vi "ADAM 5000 Get Voltages Manny.vi"(8 "error in (no error)":errorcluster, 10 "AI Sensor Data":T1={"Sensor Array"=[{"Description"="PT LOX Tank", "Last Reading"="1.37", "Coefs"=[0.0, 0.0], "Eng Units"="Psig"}, {"Description"="P3 - Fuel Tank Pressure", "Last Reading"="0.24", "Coefs"=[0.0, 5000.0], "Eng Units"="psig"}, {"Description"="P1 - Chamber Pressure", "Last Reading"="68.57", "Coefs"=[0.0, 5000.0], "Eng Units"="psig"}, {"Description"="Not Used", "Last Reading"="88.17", "Coefs"=[0.0, 0.0], "Eng Units"="psig"}, {"Description"="P5- DOME Reg.", "Last Reading"="1995.18", "Coefs"=[0.0, 5000.0], "Eng Units"="psig"}, {"Description"="Not Use", "Last Reading"="30.30", "Coefs"=[0.0, 0.0], "Eng Units"="psig"}, {"Description"="P4- High Pressure Tank", "Last Reading"="45.96", "Coefs"=[0.0, 10000.0], "Eng Units"="psig"}, {"Description"="P7 - Gnd High Pressure", "Last Reading"="1989.04", "Coefs"=[0.0, 10000.0], "Eng Units"="psig"}, {"Description"="P6 - GHE Fill Pressure", "Last Reading"="9918.82", "Coefs"=[0.0, 5000.0], "Eng Units"="psig"}, {"Description"="P8 - Pneumatics Pressure", "Last Reading"="9988.56", "Coefs"=[0.0, 5000.0], "Eng Units"="psig"}, {"Description"="Not Used", "Last Reading"="9997.25", "Coefs"=[0.0, 0.0], "Eng Units"=""}, {"Description"="Not Used", "Last Reading"="9988.56", "Coefs"=[0.0, 0.0], "Eng Units"=""}, {"Description"="Not Used", "Last Reading"="9948.58", "Coefs"=[0.0, 0.0], "Eng Units"=""}, {"Description"="Not Used", "Last Reading"="9973.45", "Coefs"=[0.0, 0.0], "Eng Units"=""}, {"Description"="Not Used", "Last Reading"="9964.45", "Coefs"=[0.0, 0.0], "Eng Units"=""}, {"Description"="PT High Press", "Last Reading"="9.16", "Coefs"=[0.0, 0.0], "Eng Units"="Psig"}, {"Description"="QD Sep Indication", "Last Reading"="2374.97", "Coefs"=[0.0, 1.0], "Eng Units"="On/Off"}, {"Description"="Lift Off Indicator", "Last Reading"="2375.24", "Coefs"=[0.0, 1.0], "Eng Units"="On/Off"}, {"Description"="Main Valve Open Indicator", "Last Reading"="2376.46", "Coefs"=[0.0, 1.0], "Eng Units"="On/Off"}, {"Description"="Main Valve Closed Indicator", "Last Reading"="2376.23", "Coefs"=[0.0, 1.0], "Eng Units"="On/Off"}, {"Description"="Load Cell 1 - Veh Gross Weight", "Last Reading"="2374.97", "Coefs"=[-122.0, 8333.3], "Eng Units"="lbf"}, {"Description"="Load Cell 2 - - Veh Gross Weight", "Last Reading"="2374.97", "Coefs"=[0.0, 8333.33], "Eng Units"="lbf"}, {"Description"="Not Used", "Last Reading"="2374.97", "Coefs"=[0.0, 0.0], "Eng Units"=""}, {"Description"="Not Used", "Last Reading"="2374.97", "Coefs"=[0.0, 0.0], "Eng Units"=""}, {"Description"="PT Fuel Tank", "Last Reading"="10.72", "Coefs"=[], "Eng Units"="Psig"}, {"Description"="", "Last Reading"="2401.98", "Coefs"=[], "Eng Units"=""}, {"Description"="PT Dome Set", "Last Reading"="0", "Coefs"=[], "Eng Units"="Psig"}, {"Description"="", "Last Reading"="2402.71", "Coefs"=[], "Eng Units"=""}, {"Description"="", "Last Reading"="2402.21", "Coefs"=[], "Eng Units"=""}, {"Description"="", "Last Reading"="2401.71", "Coefs"=[], "Eng Units"=""}, {"Description"="", "Last Reading"="2401.48", "Coefs"=[], "Eng Units"=""}, {"Description"="", "Last Reading"="2400.99", "Coefs"=[], "Eng Units"=""}]}, 11 "Remote IP Address 2":string="192.168.10.200") -> (0 "error out":errorcluster={"status"=TRUE, "code"=56, "source"="TCP Open Connection in ADAM 5000 Get Voltages Manny.vi->CalVEIN Main Manny.vi"}, 1 "Slave Input Registers 2":u16[](array[numeric]) caption="Slave Input Registers (Read Only)", 2 "Master Raw Data Vdc":dbl[](array[numeric]), 3 "AI Sensor Data Out":T1, 4 "Eng Data":dbl[](array[numeric]), 5 "Eng Data & Units":string[](array[string]))   [LabVIEW 2018]
uses:
  Adam Stuff/nimodbus121/71/vi.lib/NI Modbus.llb/MB Modbus Command.ctl
  Type Defs/Sensor Data.ctl
panel:
  out "Load Cell (lbs)":dbl=-2498.4237048905165
  out "Slave Input Registers 1":u16[](array[numeric]) caption="Slave Input Registers (Read Only)"
  out "TC Array":dbl[](array[numeric])
  out "TC String Array":string[](array[string])
  out "Test Pressure":i16
  in  "Modbus Command":T2={"Function Code"=3, "Starting Address"=0, "Quantity"=32, "Data"=[], "Discrete"=[]} {"Function Code" items=["Read Coils"=1, "Read Discrete Inputs"=2, "Read Holding Registers"=3, "Read Input Registers"=4, "Write Single Coil"=5, "Write Single Register"=6, "Read Exception Status"=7, "Write Multiple Coils"=15, "Write Multiple Registers"=16]}
  in  "Remote Port 2":u16=502
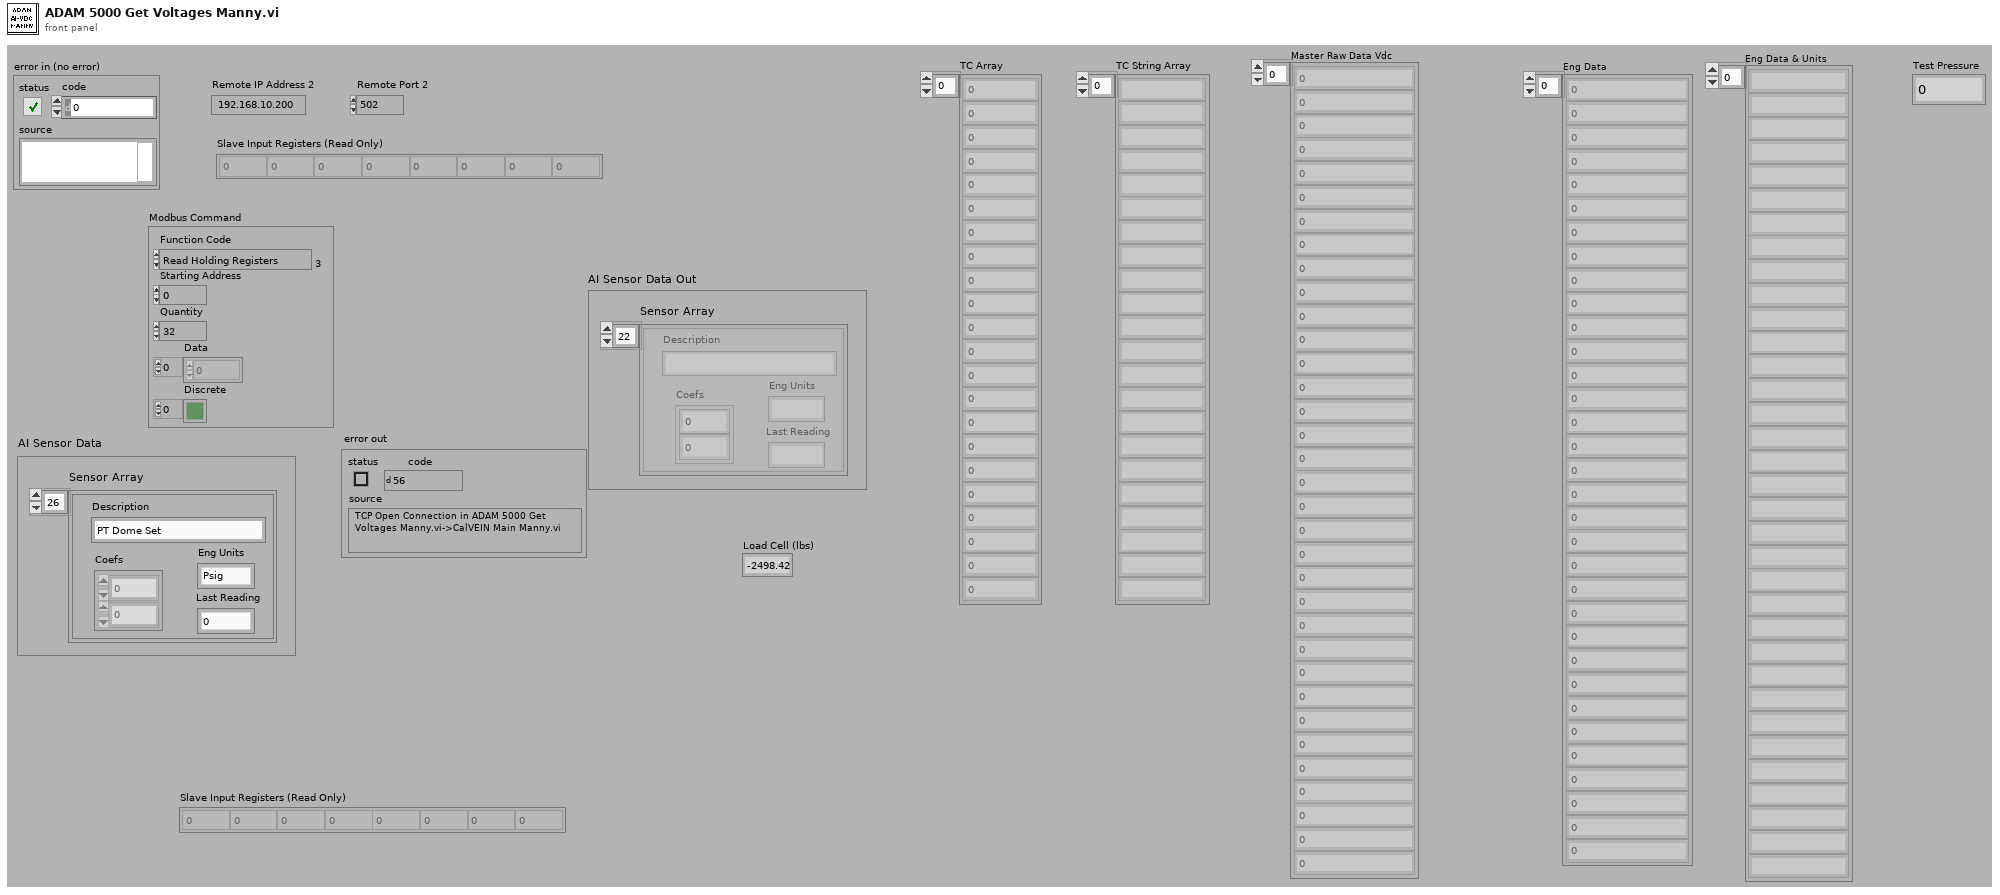
[diagram p1: front panel]
types:
  T1 = typedef "Sensor Data.ctl" = cluster{"Sensor Array":cluster{"Description":string, "Last Reading":string, "Coefs":dbl[], "Eng Units":string}[]}
  T2 = typedef "MB Modbus Command.ctl" = cluster{"Function Code":u8, "Starting Address":u16, "Quantity":u16, "Data":u16[], "Discrete":bool[]}
  T3 = cluster{"Description":string, "Last Reading":string, "Coefs":dbl[], "Eng Units":string}[]
  T4 = cluster{"Description":string, "Last Reading":string, "Coefs":dbl[], "Eng Units":string}
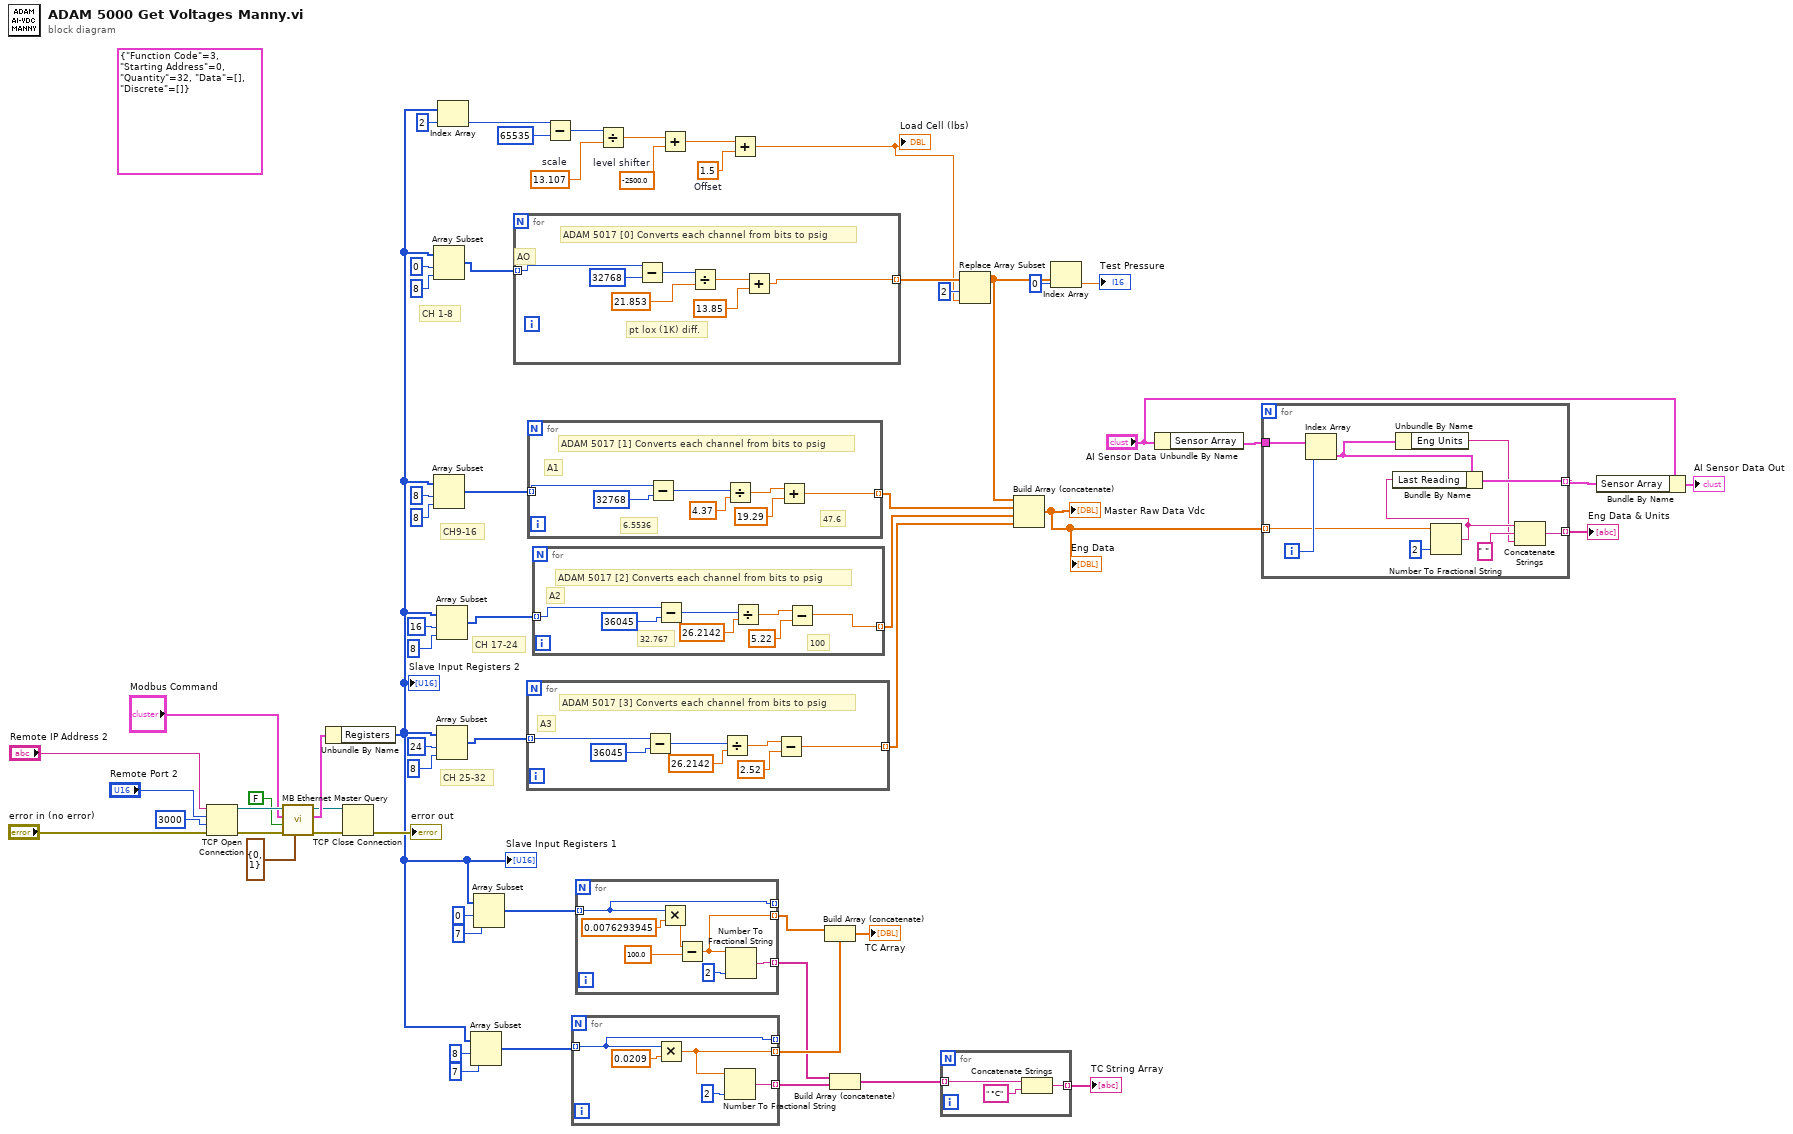
[diagram p0: block diagram]
diagram:
  w1 = 1.5  # Offset
  w10 = -2500.0  # level shifter
  w9 = 13.107  # scale
  (unwired) T2 {"Function Code"=3, "Starting Address"=0, "Quantity"=32, "Data"=[], "Discrete"=[]} ("Modbus Command")
  # "CH 25-32"
  # "CH 17-24"
  # "CH9-16"
  # "CH 1-8"
  n1 = TCP Open Connection(address="Remote IP Address 2", remote port or service name="Remote Port 2", timeout ms (60000)=3000, error in (no error)="error in (no error)") -> (connection ID=w61:refnum<k5>, error out=w55:errorcluster)  [unwired: 1 in]
  n2 = call "MB Ethernet Master Query.vi"("MBAP Header"=cluster{"Transaction ID":u16, "Unit ID":u8} {"Transaction ID"=0, "Unit ID"=1}, "error in (no error)"=w55, "Use MODBUS Data Unit?"=FALSE, "Modbus Command"="Modbus Command", "TCP Connection Refnum in"=w61) -> ("error out"=w54:errorcluster, "Registers"=w59:cluster{"Registers":u16[], "Discrete":bool[]}, "TCP Connection Refnum (dup)"=w56:refnum<k5>)  [unwired: 2 in, 2 out]
  n3 = Unbundle By Name(w59) -> ("Registers"=w13:u16[])
  "Slave Input Registers 2" <- w13
  "Slave Input Registers 1" <- w13
  n4 = TCP Close Connection(connection ID=w56, error in (no error)=w54) -> (error out=→"error out":errorcluster)  [unwired: 1 in, 1 out]
  n5 = Array Subset(array=w13, index=0, length=8) -> (w35:u16[])
  n6 = Array Subset(array=w13, index=8, length=8) -> (w48:u16[])
  n7 = Array Subset(array=w13, index=16, length=8) -> (w34:u16[])
  n8 = Array Subset(array=w13, index=24, length=8) -> (w33:u16[])
  n9 = Index Array(array=w13, index=2) -> (element=w6:u16)
  n10 = Array Subset(array=w13, index=8, length=7) -> (w19:u16[])
  n11 = Array Subset(array=w13, index=0, length=7) -> (w22:u16[])
  n12 = for {
    tunnel: w35 -> [w70] mode=indexing
    tunnel: [w69] -> w29 mode=indexing
    # "pt lox (1K) diff."
    # "AO"
    # "ADAM 5017 [0] Converts each channel from bits to psig"
    n13 = Subtract(x=w70, y=u16 32768) -> (x-y=w67:u16)
    n14 = Divide(x=w67, y=21.853) -> (x/y=w64:dbl)
    n15 = Add(x=w64, y=13.85) -> (x+y=w69:dbl)
  }
  n16 = for {
    tunnel: w33 -> [w72] mode=indexing
    tunnel: [w71] -> w27 mode=indexing
    # "A3"
    # "ADAM 5017 [3] Converts each channel from bits to psig"
    n17 = Subtract(x=w72, y=u16 36045) -> (x-y=w75:u16)
    n18 = Divide(x=w75, y=26.2142) -> (x/y=w76:dbl)
    n19 = Subtract(x=w76, y=2.52) -> (x-y=w71:dbl)
  }
  n20 = for {
    tunnel: w48 -> [w79] mode=indexing
    tunnel: [w78] -> w41 mode=indexing
    # "47.6"
    # "6.5536"
    # "A1"
    # "ADAM 5017 [1] Converts each channel from bits to psig"
    n21 = Subtract(x=w79, y=u16 32768) -> (x-y=w82:u16)
    n22 = Divide(x=w82, y=4.37) -> (x/y=w81:dbl)
    n23 = Add(x=w81, y=19.29) -> (x+y=w78:dbl)
  }
  n24 = for {
    tunnel: w34 -> [w85] mode=indexing
    tunnel: [w88] -> w32 mode=indexing
    # "A2"
    # "100"
    # "32.767"
    # "ADAM 5017 [2] Converts each channel from bits to psig"
    n25 = Subtract(x=w85, y=u16 36045) -> (x-y=w89:u16)
    n26 = Divide(x=w89, y=26.2142) -> (x/y=w87:dbl)
    n27 = Subtract(x=w87, y=5.22) -> (x-y=w88:dbl)
  }
  n28 = Subtract(x=w6, y=u16 65535) -> (x-y=w8:u16)
  n29 = for {
    tunnel: w19 -> [w92] mode=indexing
    tunnel: [w95] -> w26 mode=indexing
    tunnel: [w93] -> w24 mode=indexing
    tunnel: [w92] -> _ mode=indexing
    n30 = Multiply(x=w92, y=0.0209) -> (x*y=w95:dbl)
    n31 = Number To Fractional String(number=w95, precision (6)=i16 2) -> (F-format string=w93:string)  [unwired: 2 in]
  }
  n32 = for {
    tunnel: w22 -> [w100] mode=indexing
    tunnel: [w97] -> w25 mode=indexing
    tunnel: [w101] -> w23 mode=indexing
    tunnel: [w100] -> _ mode=indexing
    n33 = Multiply(x=w100, y=0.0076293945) -> (x*y=w99:dbl)
    n34 = Subtract(x=w99, y=100.0) -> (x-y=w97:dbl)
    n35 = Number To Fractional String(number=w97, precision (6)=i16 2) -> (F-format string=w101:string)  [unwired: 2 in]
  }
  n36 = Divide(x=w8, y=w9) -> (x/y=w11:dbl)
  n37 = Add(x=w11, y=w10) -> (x+y=w3:dbl)
  n38 = Add(x=w3, y=w1) -> (x+y=w2:dbl)
  "Load Cell (lbs)" <- w2
  n39 = Build Array (concatenate)(w25, w26) -> (→"TC Array":dbl[])
  n40 = Build Array (concatenate)(w23, w24) -> (w15:string[])
  n41 = for {
    tunnel: w15 -> [w106] mode=indexing
    tunnel: [w104] -> w16 mode=indexing
    n42 = Concatenate Strings(w106, " °C") -> (w104:string)
  }
  "TC String Array" <- w16
  n43 = Replace Array Subset(array=w29, new element=w2, index=2) -> (w5:dbl[])
  n44 = Build Array (concatenate)(w5, w41, w32, w27) -> (w28:dbl[])
  "Master Raw Data Vdc" <- w28
  "Eng Data" <- w28
  n45 = Index Array(array=w5, index=0) -> (element=→"Test Pressure":dbl)
  n46 = Unbundle By Name("AI Sensor Data") -> ("Sensor Array"=w40:T3)
  n47 = for {
    tunnel: w40 -> [w116]
    tunnel: w28 -> [w107] mode=indexing
    tunnel: [w112] -> w38 mode=indexing
    tunnel: [w108] -> w36 mode=indexing
    i -> [w115]
    n48 = Index Array(array=w116, index=w115) -> (element=w114:T4)
    n49 = Unbundle By Name(w114) -> ("Eng Units"=w109:string)
    n50 = Number To Fractional String(number=w107, precision (6)=i16 2) -> (F-format string=w111:string)  [unwired: 2 in]
    n51 = Bundle By Name(cluster=w114, "Last Reading"=w111) -> (w112:T4)
    n52 = Concatenate Strings(w111, " " ("string"), w109) -> (w108:string)
  }
  "Eng Data & Units" <- w36
  n53 = Bundle By Name(cluster="AI Sensor Data", "Sensor Array"=w38) -> (→"AI Sensor Data Out":T1)
